vi "Ctor.vi"(8 "error in (no error)":errorcluster, 9 "TCP Port":u16=4763, 10 "WS Port":u16, 11 "HTTP Port":u16) -> (0 "error out":errorcluster, 3 "LV Server out":refnum<class "LV Server.lvclass">)   [LabVIEW 2020, in "LV Server.lvclass"]
uses:
  LV Server.lvclass
  LV Server.lvclass/LV Server.ctl
  Timer Data.ctl
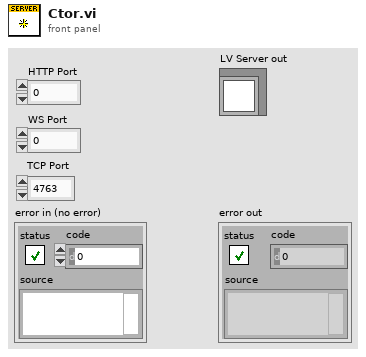
[diagram p1: front panel]
types:
  T1 = typedef "LV Server.lvclass/Timer Data.ctl" = cluster{"Start":dbl, "Accumulated":dbl, "Running":bool}
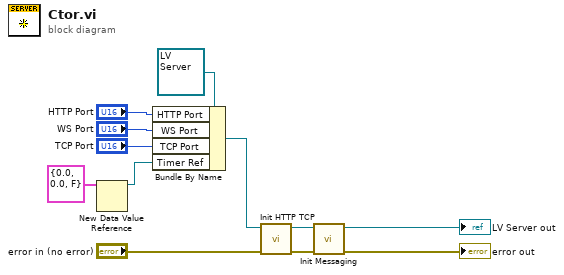
[diagram p0: block diagram]
diagram:
  n1 = New Data Value Reference(data value=T1 {"Start"=0.0, "Accumulated"=0.0, "Running"=FALSE} ("Timer Data")) -> (data value reference=w6:refnum<data-value>)  [unwired: 1 in, 1 out]
  n2 = Bundle By Name(cluster=refnum<class "LV Server.lvclass"> refnum ("LV Server in"), "HTTP Port"="HTTP Port", "WS Port"="WS Port", "TCP Port"="TCP Port", "Timer Ref"=w6) -> (w8:refnum<class "LV Server.lvclass">)
  n3 = call "Init HTTP TCP.vi"("error in (no error)"="error in (no error)", "LV Server in"=w8) -> ("error out"=w4:errorcluster, "LV Server out"=w5:refnum<class "LV Server.lvclass">)  [unwired: 8 in]
  n4 = call "Init Messaging.vi"("error in (no error)"=w4, "LV Server in"=w5) -> ("error out"=→"error out":errorcluster, "LV Server out"=→"LV Server out":refnum<class "LV Server.lvclass">)  [unwired: 8 in]
